vi "TestMain.vi"() -> ()   [LabVIEW 2019]
uses:
  <vilib>/Platform/TimedLoop/XDataNode/timing_clust.ctl
  <vilib>/Platform/TimedLoop/XDataNode/nitl_modes.ctl
  <vilib>/Platform/TimedLoop/XDataNode/wakeup.ctl
  <vilib>/myRIO/Instrument Drivers/Onboard IO/PWM/typedefs/PWM Reference.ctl
  <vilib>/myRIO/Common/Instrument Driver Framework/Utilities/typedefs/myRIO Generic Hardware Reference.ctl
  <vilib>/myRIO/Common/Instrument Driver Framework/Utilities/typedefs/Hardware Version Enum.ctl
  <vilib>/myRIO/Common/Instrument Driver Framework/Utilities/typedefs/myRIO v1.0 Reference.ctl
  <vilib>/myRIO/Common/Instrument Driver Framework/Utilities/typedefs/Generic FPGA Reference.ctl
  <vilib>/myRIO/Common/Instrument Driver Framework/myRIO v1.0/PWM/typedefs/PWM Channels Enum.ctl
  <vilib>/myRIO/Instrument Drivers/Onboard IO/PWM/typedefs/PWM Configuration.ctl
  <vilib>/userDefined/High Color/nirio_resource_hc.ctl
  <vilib>/myRIO/Instrument Drivers/Onboard IO/DIO/typedefs/DIO Reference.ctl
  <vilib>/myRIO/Common/Instrument Driver Framework/myRIO v1.0/DIO/typedefs/DIO Channels List.ctl
  <vilib>/myRIO/Common/Instrument Driver Framework/myRIO v1.0/DIO/typedefs/DIO Channels Enum.ctl
  <vilib>/myRIO/Common/Instrument Driver Framework/Utilities/vis/Is FPGA Ref Available.vi
  <vilib>/myRIO/Common/Instrument Driver Framework/myRIO v1.0/PWM/vis/myRIO v1.1 Open PWM.vi
  <vilib>/myRIO/Instrument Drivers/Onboard IO/PWM/vis/Set Duty Cycle and Frequency.vi
  <vilib>/myRIO/Common/Instrument Driver Framework/myRIO v1.0/DIO/vis/myRIO v1.1 Open DIO.vi
  <extravilib>/ChannelInstances/Tag-bool/Write With Abort.vi
  <extravilib>/ChannelInstances/Tag-bool/Read With Abort.vi
  <vilib>/myRIO/Common/Instrument Driver Framework/Utilities/vis/Validate Channels.vi
  <vilib>/myRIO/Common/Instrument Driver Framework/myRIO v1.0/PWM/vis/myRIO v1.0 Reserve PWM.vi
  <vilib>/myRIO/Common/Instrument Driver Framework/myRIO v1.0/DIO/vis/myRIO v1.0 Reserve DIO.vi
  <vilib>/myRIO/Common/Instrument Driver Framework/myRIO v1.0/I2C/vis/myRIO v1.0 Close I2C.vi
  <vilib>/myRIO/Common/Instrument Driver Framework/myRIO v1.0/UART/vis/myRIO v1.0 Close UART.vi
  <vilib>/myRIO/Common/Instrument Driver Framework/myRIO v1.0/PWM/vis/myRIO v1.0 Build MUX Configuration PWM.vi
  <vilib>/myRIO/Common/Instrument Driver Framework/myRIO v1.0/Resource Manager/vis/myRIO v1.0 Reserve Channel List.vi
  <vilib>/myRIO/Common/Instrument Driver Framework/myRIO v1.0/DIO/vis/myRIO v1.0 Build MUX Configuration DIO.vi
  <vilib>/myRIO/Common/Instrument Driver Framework/myRIO v1.0/I2C/vis/myRIO v1.0 Unreserve I2C.vi
  <vilib>/myRIO/Common/Instrument Driver Framework/myRIO v1.0/Resource Manager/vis/myRIO v1.0 Create Configuration List.vi
  <vilib>/myRIO/Common/Instrument Driver Framework/myRIO v1.0/Resource Manager/vis/myRIO v1.0 Reserve Channel.vi
  <vilib>/myRIO/Common/Instrument Driver Framework/myRIO v1.0/Resource Manager/vis/myRIO v1.0 Unreserve Channel.vi
  <vilib>/myRIO/Common/Instrument Driver Framework/myRIO v1.0/I2C/vis/myRIO v1.0 Build MUX Configuration I2C.vi
  <vilib>/myRIO/Common/Instrument Driver Framework/myRIO v1.0/Resource Manager/vis/myRIO v1.0 Unreserve Channel List.vi
  <vilib>/myRIO/Common/Instrument Driver Framework/myRIO v1.0/Resource Manager/vis/myRIO v1.0 Build Mutex Name.vi
  <extravilib>/ChannelInstances/Tag-bool/Instantiate.vi
  <extravilib>/ChannelInstances/Tag-bool/EndpointRead.vi
  <vilib>/Utility/VariantDataType/GetNumericInfo.vi
  <vilib>/Utility/error.llb/Error Cluster From Error Code.vi
  <vilib>/myRIO/Common/Instrument Driver Framework/myRIO v1.0/myRIO v1.1 Open.vi
  <vilib>/myRIO/Common/Instrument Driver Framework/Utilities/vis/IO Manager.vi
  <vilib>/myRIO/Common/Instrument Driver Framework/Utilities/vis/Configuration Manager.vi
  <vilib>/myRIO/Common/Instrument Driver Framework/myRIO v1.0/Resource Manager/vis/myRIO v1.0 Configure IO.vi
  <vilib>/myRIO/Common/Instrument Driver Framework/myRIO v1.0/myRIO v1.0 Close.vi
  <vilib>/myRIO/Common/Instrument Driver Framework/myRIO v1.0/PWM/vis/myRIO v1.0 Write PWM.vi
  <vilib>/myRIO/Common/Instrument Driver Framework/myRIO v1.0/DIO/vis/myRIO v1.0 Write DIO.vi
  <vilib>/myRIO/Common/Instrument Driver Framework/myRIO v1.0/I2C/vis/myRIO v1.0 Shutdown I2C.vi
  <vilib>/rvi/errors/niLvFpgaAdjustHostInterfaceError.vi
  <vilib>/FPGAPlugInAG/Dynamic/niLvFpga_Abort_Dynamic.vi
  <vilib>/myRIO/Common/Instrument Driver Framework/Utilities/vis/FPGA Ref Manager.vi
  <vilib>/myRIO/Common/Instrument Driver Framework/myRIO v1.0/myRIO v1.0 Reset FPGA.vi
  <vilib>/myRIO/Common/Instrument Driver Framework/myRIO v1.0/IRQ/vis/myRIO v1.0 IRQ Info FGV.vi
  <vilib>/myRIO/Common/Instrument Driver Framework/myRIO v1.0/IRQ/vis/myRIO v1.0 Timer IRQ Info FGV.vi
  <vilib>/myRIO/Common/Instrument Driver Framework/myRIO v1.0/IRQ/vis/myRIO v1.0 ISR Agent.vi
  <vilib>/myRIO/Instrument Drivers/Utilities/vis/Reset Index.vi
  <vilib>/myRIO/Common/Instrument Driver Framework/myRIO v1.0/Resource Manager/vis/myRIO v1.0 Block Write Resource Manager.vi
  <vilib>/FPGAPlugInAG/Dynamic/niLvFpga_Close_Dynamic.vi
  <extravilib>/ChannelInstances/Tag-bool/Endpoint.vi
  <vilib>/platform/TimedLoop/XDataNode/XDataNode.xnode
  <vilib>/myRIO/Express VI/Onboard IO/PWM/PWM Express VI.xnode
  <vilib>/myRIO/Instrument Drivers/Onboard IO/PWM/vis/myRIO PWM Open.xnode
  <vilib>/myRIO/Express VI/Onboard IO/DO/DO Express VI.xnode
  <vilib>/myRIO/Instrument Drivers/Onboard IO/DIO/vis/myRIO DIO Open.xnode
  <vilib>/rvi/interface/nirviReadWriteControl/nirviReadWriteControl.xnode
  <vilib>/rvi/interface/nirviMethod/nirviMethod.xnode
  <vilib>/rvi/interface/nirviCloseFPGA/nirviCloseFPGA.xnode
  <vilib>/rvi/interface/Simulation/niFpgaSimulationCallBeginRW.vi
  <vilib>/Platform/TimedLoop/XDataNode/XDNodeRunTimeDep.lvlib
  <vilib>/myRIO/Instrument Drivers/Utilities/Utilities.lvlib
  NiFpgaLv.dll
  <extravilib>/ChannelInstances/Tag-bool.lvlib
  <vilib>/myRIO/Instrument Drivers/Onboard IO/PWM/PWM.lvlib
  <vilib>/myRIO/Instrument Drivers/Onboard IO/DIO/DIO.lvlib
  <vilib>/myRIO/Instrument Drivers/Onboard IO/I2C/I2C.lvlib
panel:
  in  "Speed (km/h)":dbl
  in  "Test FM only":bool
  in  "Old (F), new (T) PID":bool
  in  "Inner PID T/F":bool
  in  "D_i":dbl
  in  "I_i":dbl
  in  "P_i":dbl
  in  "Log file path":path
  out "Duty Cycle":dbl
  in  "Angle limit":i32
  in  "D_o":dbl
  in  "I_o":dbl
  in  "P_o":dbl
  out "Combined loop duration time (us)":i64
  in  "Loop durations":T1(tab)
  out "IMU Data gathering duration(us)":i64(graph)
  out "Encoder data gathering duration(us)":i64(graph)
  out "Steering Motor duration(us)":i64(graph)
  out "E-Stop loop duration (us)":i64(graph)
  in  "GO":bool
  in  "E-stop":bool
  out "Indicator":bool
  in  "Encoder Position Reset":bool
  out "Encoder Velocity (Counts/Interval)":i32
  out "Encoder Acceleration (Counts/Interval)":i32
  out "Encoder Position (Counts)":i32
  out "IMU Gyro Chart":cluster{dbl, dbl, dbl}(graph)
  out "IMU Acc Chart":cluster{dbl, dbl, dbl}(graph)
  # "Steering Motor"
  # "Forward Motor"
  # "Outer"
  # "Inner"
  # "Start Motors"
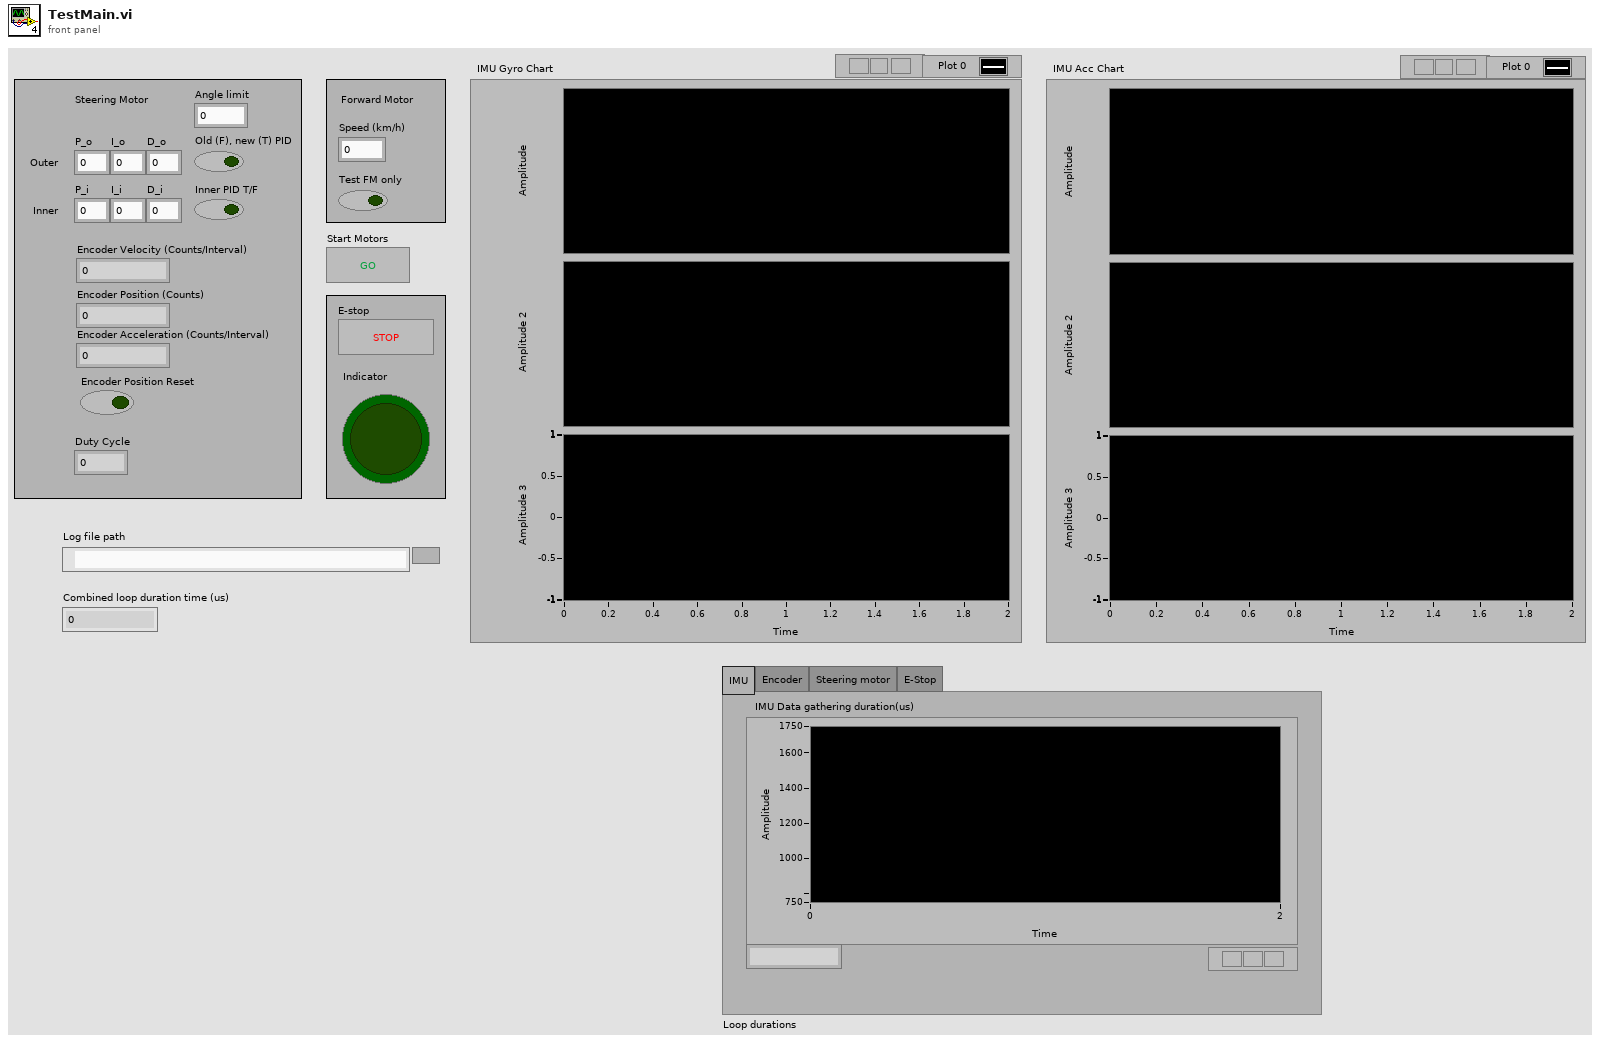
[diagram p1: front panel]
types:
  T1 = enum32{"IMU", "Encoder", "Steering motor", "E-Stop"}
  T2 = enum16{"open", "open or create", "create or replace", "create", "open (read-only)"}
  T3 = typedef "I2C.lvlib/I2C Reference.ctl" = cluster{"myRIO Reference":T4, "I2C Channels Enum":T8, "I2C Configuration":T9}
  T4 = typedef "myRIO Generic Hardware Reference.ctl" = cluster{"myRIO Model":T5, "myRIO Hardware Reference":T6}
  T5 = typedef "Hardware Version Enum.ctl" = enum16{"Unknown", "myRIO-1900", "myRIO-1950", "roboRIO", "NI ELVIS RIO CM", "ELVIS III"}
  T6 = typedef "myRIO v1.0 Reference.ctl" = cluster{"Generic FPGA Reference":T7, "Allow multiple opens":bool}
  T7 = typedef "Generic FPGA Reference.ctl" = refnum<k20>
  T8 = typedef "I2C Channels Enum.ctl" = enum16{"Not Connected", "A/I2C", "B/I2C", "I2C/I2C"}
  T9 = typedef "I2C.lvlib/I2C Configuration.ctl" = cluster{"I2C Transfer Rate":T10}
  T10 = typedef "I2C.lvlib/I2C Transfer Rate.ctl" = enum16{"Standard mode (100 kbps)", "Fast mode (400 kbps)"}
  T11 = typedef "XDNodeRunTimeDep.lvlib/timing_clust.ctl" = cluster{"Expected End [f-1]":u64, "Actual End [f-1]":u64, "Finished Late? [f-1]":bool, "Expected End [i-1]":u64, "Actual End [i-1]":u64, "Finished Late? [i-1]":bool, "Expected Start [i]":u64, "Actual Start [i]":u64, "Expected Start [f]":u64, "Actual Start [f]":u64, "Source Name":string, "Structure Name":string, "Period":i64, "Deadline":i64, "Offset":i64, "Start":i64, "Priority":i32, "Timeout":i32, "Mode":T12, "Wakeup Reason":T13, "Error":errorcluster, "Source Type":string, "Secondary Source Type":string, "Global End Time":u64, "Global Start Time":u64, "Frame Duration":u64, "Iteration Duration":u64, "Assigned CPU":i32, "I/O Scan Engine Mode":u32}
  T12 = typedef "XDNodeRunTimeDep.lvlib/nitl_modes.ctl" = enum32{"No Change", "Process missed periods, maintain original phase", "Discard missed periods, maintain original phase", "Process missed periods, ignore original phase", "Discard missed periods, ignore original phase"}
  T13 = typedef "XDNodeRunTimeDep.lvlib/wakeup.ctl" = enum32{"Normal", "Aborted", "Asynchronous wakeup", "Timing source error", "Timed loop error", "Timeout"}
  T14 = typedef "Tag-bool.lvlib/))Channel.ctl" = refnum<queue>
  T15 = typedef "PWM.lvlib/PWM Reference.ctl" = cluster{"myRIO Reference":T4, "PWM Channels Enum":T16, "PWM Configuration":T17}
  T16 = typedef "PWM Channels Enum.ctl" = enum16{"Not Connected", "C/PWM0", "C/PWM1", "A/PWM0", "A/PWM1", "A/PWM2", "A/PWM3", "A/PWM4", "A/PWM5", "A/PWM6", "A/PWM7", "A/PWM8", "A/PWM9", "A/PWM10", "A/PWM11", "A/PWM12", "A/PWM13", "A/PWM14", "A/PWM15", "A/PWM16", "A/PWM17", "A/PWM18", "A/PWM19", "B/PWM0", "B/PWM1", "B/PWM2", "B/PWM3", "B/PWM4", "B/PWM5", "B/PWM6", "B/PWM7", "B/PWM8", "B/PWM9", "B/PWM10", "B/PWM11", "B/PWM12", "B/PWM13", "B/PWM14", "B/PWM15", "B/PWM16", "B/PWM17", "B/PWM18", "B/PWM19", "PWM/PWM0", "PWM/PWM1", "PWM/PWM2", "PWM/PWM3", "PWM/PWM4", "PWM/PWM5", "PWM/PWM6", "PWM/PWM7", "PWM/PWM8", "PWM/PWM9"}
  T17 = typedef "PWM.lvlib/PWM Configuration.ctl" = cluster{"Frequency":dbl, "Duty Cycle":dbl}
  T18 = typedef "nirio_resource_hc.ctl" = tag
  T19 = typedef "DIO.lvlib/DIO Reference.ctl" = cluster{"myRIO Reference":T4, "DIO Channels List":T20}
  T20 = typedef "DIO Channels List.ctl" = T21[]
  T21 = typedef "DIO Channels Enum.ctl" = enum16{"Not Connected", "C/DIO0", "C/DIO1", "C/DIO2", "C/DIO3", "C/DIO4", "C/DIO5", "C/DIO6", "C/DIO7", "A/DIO0", "A/DIO1", "A/DIO2", "A/DIO3", "A/DIO4", "A/DIO5", "A/DIO6", "A/DIO7", "A/DIO8", "A/DIO9", "A/DIO10", "A/DIO11", "A/DIO12", "A/DIO13", "A/DIO14", "A/DIO15", "A/DIO16", "A/DIO17", "A/DIO18", "A/DIO19", "B/DIO0", "B/DIO1", "B/DIO2", "B/DIO3", "B/DIO4", "B/DIO5", "B/DIO6", "B/DIO7", "B/DIO8", "B/DIO9", "B/DIO10", "B/DIO11", "B/DIO12", "B/DIO13", "B/DIO14", "B/DIO15", "B/DIO16", "B/DIO17", "B/DIO18", "B/DIO19", "LED0", "LED1", "LED2", "LED3", "Button0", "DIO/DIO0", "DIO/DIO1", "DIO/DIO2", "DIO/DIO3", "DIO/DIO4", "DIO/DIO5", "DIO/DIO6", "DIO/DIO7", "DIO/DIO8", "DIO/DIO9", "SPI/CS0", "SPI/CS1", "SPI/CS2", "SPI/CS3", "LED RADIO (Green)", "LED RADIO (Red)", "LED COMM (Green)", "LED COMM (Red)", "LED MODE (Green)", "LED MODE (Red)"}
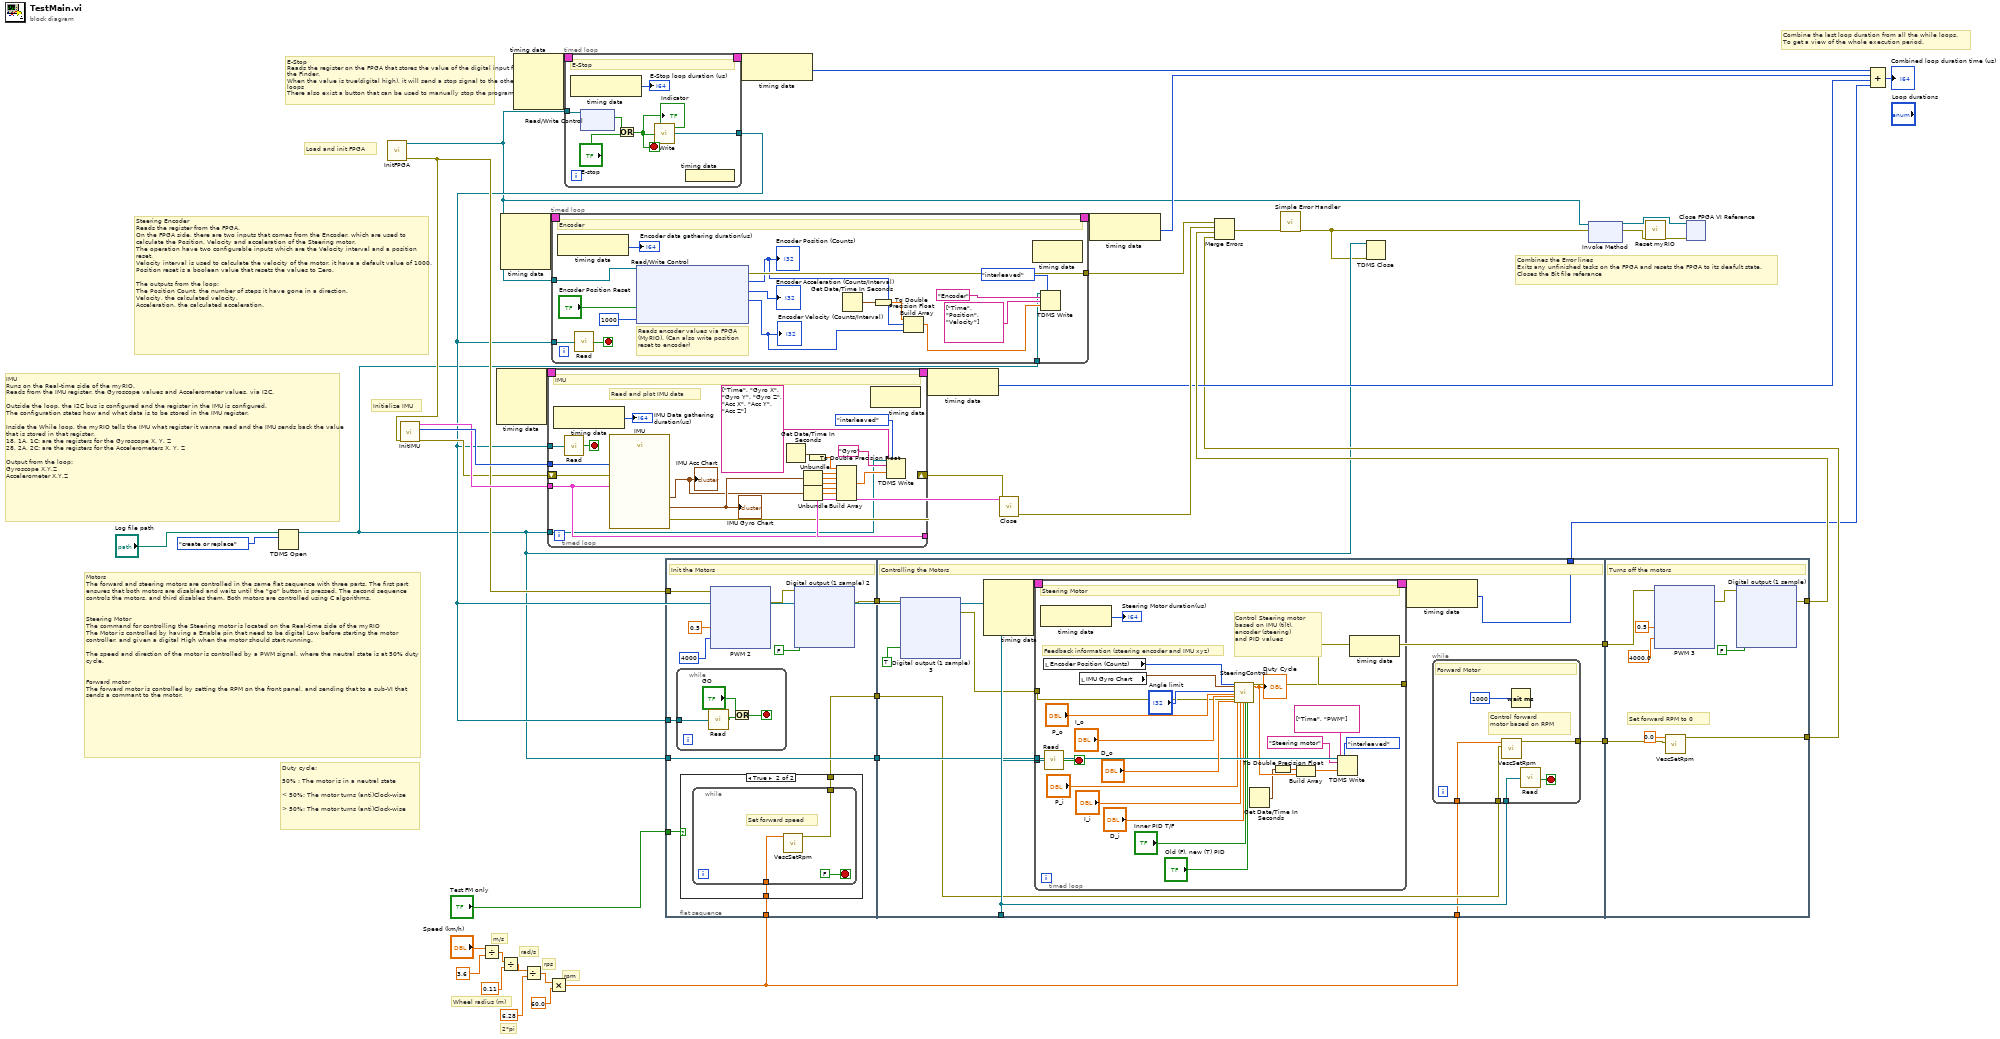
[diagram p0: block diagram]
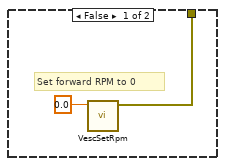
[diagram p2: hidden frame]
diagram:
  # "2*pi"
  # "rpm"
  # "rps"
  # "rad/s"
  # "Wheel radius (m)"
  # "m/s"
  # "Duty cycle:\n\n50% : The motor is in a neutral state\n\n< 50%: The motor turns (anti)Clock-wise\n\n> 50%: The motor turns (anti)Clock-wise"
  # "Initialize IMU"
  # "Load and init FPGA"
  # "Combines the Error lines\nExits any unfinished tasks on the FPGA and resets the FPGA to its deafult state.\nCloses the Bit file referance"
  # "Combine the last loop duration from all the while loops.\nTo get a view of the whole execution period."
  # "Motors\nThe forward and steering motors are controlled in the same flat sequence with three parts. The first part ensures that both motors are disabled and waits until the \"go\" button is pressed. The second sequence controls the motors, and third disables them. Both motors are controlled using C algorithms.\n\n\nSteering Motor\nThe command for controlling the Steering motor is located on the Real-time side of the myRIO\nThe Motor is controlled by having a Enable pin that need to be digital Low before starting the motor controller, and given a digital High when the motor should start running.\n\nThe speed and direction of the motor is controlled by a PWM signal, where the neutral state is at 50% duty cycle.\n\n\nForward motor\nThe forward motor is controlled by setting the RPM on the front panel, and sending that to a sub-VI that sends a commant to the motor."
  # "IMU\nRuns on the Real-time side of the myRIO.\nReads from the IMU register, the Gyroscope values and Accelerometer values, via I2C.\n\nOutside the loop, the I2C bus is configured and the register in the IMU is configured.\nThe configuration states how and what data is to be stored in the IMU register.\n\nInside the While loop, the myRIO tells the IMU what register it wanna read and the IMU sends back the value that is stored in that register.\n18, 1A, 1C: are the registers for the Gyroscope X, Y, Z\n28, 2A, 2C: are the registers for the Accelerometers X, Y, Z\n\nOutput from the loop:\nGyroscope X,Y,Z\nAccelerometer X,Y,Z"
  # "Steering Encoder\nReads the register from the FPGA. \nOn the FPGA side, there are two inputs that comes from the Encoder, which are used to calculate the Position, Velocity and acceleration of the Steering motor.\nThe operation have two configurable inputs which are the Velocity interval and a position reset.\nVelocity interval is used to calculate the velocity of the motor, it have a default value of 1000.\nPosition reset is a boolean value that resets the values to Zero.\n\nThe outputs from the loop:\nThe Position Count, the number of steps it have gone in a direction. \nVelocity, the calculated velocity.\nAcceleration, the calculated acceleration."
  # "E-Stop\nReads the register on the FPGA that stores the value of the digital input from the Finder.\nWhen the value is true(digital high), it will send a stop signal to the other while loops\nThere also exist a button that can be used to manually stop the program."
  n1 = TDMS Open(10:T2."create or replace" ("operation (0:open)"), 11:"Log file path") -> (3:w15:refnum<k34>)  [unwired: 5 in, 1 out]
  n2 = call "InitFPGA.vi"() -> ("error out"=w30:errorcluster, "Refnum out"=w11:refnum<k20>)  [unwired: 10 in]
  n3 = call "InitIMU.vi"("error in (no error)"=w30) -> ("error out"=w25:errorcluster, "Acc/Gyro  address"=w32:u8, "I2C Ref Out"=w31:T3)  [unwired: 8 in]
  n4 = Divide(x="Speed (km/h)", y=3.6) -> (x/y=w7:dbl)
  n5 = node-c288() -> (w39:T11)  [unwired: 4 in]
  n6 = node-c288() -> (w43:T11)  [unwired: 4 in]
  n7 = Divide(x=w7, y=0.11) -> (x/y=w5:dbl)
  n8 = node-c288() -> (w37:T11)  [unwired: 4 in]
  n9 = Divide(x=w5, y=6.28) -> (x/y=w4:dbl)
  n10 = Multiply(x=w4, y=60.0) -> (x*y=w1:dbl)
  n11 = timed-loop {
    timing: w37 -> [_]
    timing-out: [_] -> w36
    tunnel: w11 -> [w52]
    tunnel: [w51] -> w23
    stop <- w47 stop-if-true
    # "E-Stop"
    n12 = node-c288() -> (→"E-Stop loop duration (us)":i64)  [unwired: 1 in]
    n13 = xnode "Read/Write Control"("FPGA VI Reference In"=w52) -> ("E-Stop"=w50:bool)  [unwired: 1 in, 2 out]
    n14 = Or(x=w50, y="E-stop") -> (x .or. y?=w47:bool)
    "Indicator" <- w47
    n15 = call <vilib>:"Write.vi"("element"=w47) -> ("channel"=w51:T14)  [unwired: 1 out]
    n16 = node-c288() -> ()  [unwired: 1 out]
  }
  n17 = timed-loop {
    timing: w39 -> [_]
    timing-out: [_] -> w38
    tunnel: w32 -> [w77]
    tunnel: w31 -> [w74]
    shift-right: [w71] -> w26
    shift-left: w25 -> [w76]
    tunnel: [w74] -> w29
    tunnel: w23 -> [w73]
    tunnel: w15 -> [w66]
    stop <- w72 stop-if-true
    # "Read and plot IMU data"
    # "IMU"
    n18 = node-c288() -> (→"IMU Data gathering duration(us)":i64)  [unwired: 1 in]
    n19 = call <extravilib>:"Read.vi"("channel"=w73) -> ("element"=w72:bool)  [unwired: 1 in, 1 out]
    n20 = call "IMU.vi"("error in (no error)"=w76, "Acc/Gyro  address"=w77, "I2C Ref"=w74) -> ("error out"=w71:errorcluster, "IMU Acc"=w59:cluster{dbl, dbl, dbl}, "IMU Gyro"=w70:cluster{dbl, dbl, dbl})  [unwired: 6 in]
    "IMU Acc Chart" <- w59
    "IMU Gyro Chart" <- w70
    n21 = Get Date/Time In Seconds() -> (seconds since 1Jan1904=w64:timestamp)
    n22 = Unbundle(w70) -> (w69:dbl, w61:dbl, w60:dbl)
    n23 = Unbundle(w59) -> (w58:dbl, w57:dbl, w56:dbl)
    n24 = To Double Precision Float(number=w64) -> (double precision float=w65:dbl)
    n25 = Build Array(w65, w69, w61, w60, w58, w57, w56) -> (w67:dbl[])
    n26 = node-c288() -> ()  [unwired: 1 in, 1 out]
    n27 = TDMS Write(0:w66, 1:enum16{"decimated", "interleaved"}."interleaved" ("data layout (0:decimated)"), 5:"Gyro" ("group name in (Untitled)"), 7:string[] ["Time", "Gyro X", "Gyro Y", "Gyro Z", "Acc X", "Acc Y", "Acc Z"] ("channel name(s) in (Untitled)"), 9:w67) -> ()  [unwired: 1 in, 4 out]
  }
  n28 = timed-loop {
    timing: w43 -> [_]
    timing-out: [_] -> w42
    tunnel: w11 -> [w97]
    tunnel: [w96] -> w41
    tunnel: w23 -> [w91]
    tunnel: w15 -> [w84]
    stop <- w90 stop-if-true
    # "Reads encoder values via FPGA\n(MyRIO). (Can also write position\nreset to encoder)"
    # "Encoder"
    n29 = node-c288() -> (→"Encoder data gathering duration(us)":i64)  [unwired: 1 in]
    n30 = call <extravilib>:"Read.vi"("channel"=w91) -> ("element"=w90:bool)  [unwired: 1 in, 1 out]
    n31 = xnode "Read/Write Control"("FPGA VI Reference In"=w97, "Position Reset"="Encoder Position Reset", "Velocity Interval (uSec)"=u32 1000) -> ("error out"=w96:errorcluster, "Position (Counts)"=w87:i32, "Acceleration (Counts/Interval)"=→"Encoder Acceleration (Counts/Interval)":i32, "Velocity (Counts/Interval)"=w86:i32)  [unwired: 1 in, 1 out]
    "Encoder Position (Counts)" <- w87
    "Encoder Velocity (Counts/Interval)" <- w86
    n32 = Get Date/Time In Seconds() -> (seconds since 1Jan1904=w82:timestamp)
    n33 = To Double Precision Float(number=w82) -> (double precision float=w83:dbl)
    n34 = Build Array(w83, w87, w86) -> (w85:dbl[])
    n35 = node-c288() -> ()  [unwired: 1 in, 1 out]
    n36 = TDMS Write(0:w84, 1:enum16{"decimated", "interleaved"}."interleaved" ("data layout (0:decimated)"), 5:"Encoder" ("group name in (Untitled)"), 7:string[] ["Time", "Position", "Velocity"] ("channel name(s) in (Untitled)"), 9:w85) -> ()  [unwired: 1 in, 4 out]
  }
  n37 = flat-sequence {
    tunnel: [w110] -> w35
    tunnel: w30 -> [w108]
    tunnel: w23 -> [w105]
    tunnel: [w101] -> w22
    tunnel: w15 -> [w104]
    tunnel: [w104] -> w16
    tunnel: "Test FM only" -> [w103]
    tunnel: w1 -> [w102]
    tunnel: w35 -> [w204]
    tunnel: [w201] -> w13
    tunnel: w23 -> [w198]
    tunnel: w22 -> [w194]
    tunnel: [w197] -> w21
    tunnel: [w196] -> w19
    tunnel: w16 -> [w195]
    tunnel: w1 -> [w193]
    tunnel: [w283] -> w27
    tunnel: w21 -> [w278]
    tunnel: [w277] -> w20
    tunnel: w19 -> [w276]
    frame #0 {
      # "Init the Motors"
      n38 = while {
        tunnel: w105 -> [w119]
        stop <- w122 stop-if-true
        n39 = call <extravilib>:"Read.vi"("channel"=w119) -> ("element"=w120:bool)  [unwired: 1 in, 1 out]
        n40 = Or(x="GO", y=w120) -> (x .or. y?=w122:bool)
      }
      n41 = case shown="True" w103 {
        tunnel: w102 -> [_ w115]
        tunnel: [w112 w114] -> w101
        frame False {
          # "Set forward RPM to 0"
          n42 = call "VescSetRpm.vi"("Speed (rpm)"=0.0) -> ("error out"=w112:errorcluster)  [unwired: 10 in]
        }
        frame True {
          n43 = while {
            tunnel: w115 -> [w118]
            tunnel: [w116] -> w114
            stop <- FALSE stop-if-true
            # "Set forward speed"
            n44 = call "VescSetRpm.vi"("Speed (rpm)"=w118) -> ("error out"=w116:errorcluster)  [unwired: 10 in]
          }
        }
      }
      n45 = xnode "PWM 2"("Duty Cycle"=0.5, "Frequency [Hz]"=4000, "error in (no error)"=w108) -> ("error out"=w111:errorcluster)
      n46 = xnode "Digital output (1 sample) 2"("B/DIO4 (Pin 19)"=FALSE ("B/DIO1 (Pin 13)"), "error in (no error)"=w111) -> ("error out"=w110:errorcluster)
    }
    frame #1 {
      # "Controlling the Motors"
      n47 = xnode "Digital output (1 sample) 3"("B/DIO4 (Pin 19)"=TRUE ("B/DIO1 (Pin 13)"), "error in (no error)"=w204) -> ("error out"=w200:errorcluster)
      n48 = node-c288() -> (w203:T11)  [unwired: 4 in]
      n49 = timed-loop {
        tunnel: w200 -> [w225]
        timing: w203 -> [_]
        timing-out: [_] -> w202
        tunnel: w198 -> [w227]
        tunnel: [w224] -> w196
        tunnel: w195 -> [w223]
        stop <- w234 stop-if-true
        # "Feedback information (steering encoder and IMU xyz)"
        # "Control Steering motor\nbased on IMU (tilt), \nencoder (steering)\nand PID values"
        # "Steering Motor"
        n50 = node-c288() -> (→"Steering Motor duration(us)":i64)  [unwired: 1 in]
        n51 = local read "Encoder Position (Counts)"() -> (w231:i32)
        n52 = call <extravilib>:"Read.vi"("channel"=w227) -> ("element"=w234:bool)  [unwired: 1 in, 1 out]
        n53 = local read "IMU Gyro Chart"() -> (w232:cluster{dbl, dbl, dbl})
        n54 = call "SteeringControl.vi"("Position (Counts)"=w231, "Cluster"=w232, "Limit"="Angle limit", "P_o gain"="P_o", "I_o gain"="I_o", "error in (no error)"=w225, "D_o gain"="D_o", "P_i gain"="P_i", "I_i gain"="I_i", "D_i gain"="D_i", "Inner PID T/F"="Inner PID T/F", "Old (F), new (T) PID"="Old (F), new (T) PID") -> ("error out"=w224:errorcluster, "PWM Out"=w220:dbl)  [unwired: 14 in]
        "Duty Cycle" <- w220
        n55 = Get Date/Time In Seconds() -> (seconds since 1Jan1904=w218:timestamp)
        n56 = To Double Precision Float(number=w218) -> (double precision float=w219:dbl)
        n57 = Build Array(w219, w220) -> (w221:dbl[])
        n58 = TDMS Write(0:w223, 1:enum16{"decimated", "interleaved"}."interleaved" ("data layout (0:decimated)"), 5:"Steering motor" ("group name in (Untitled)"), 7:string[] ["Time", "PWM"] ("channel name(s) in (Untitled)"), 9:w221) -> ()  [unwired: 1 in, 4 out]
        n59 = node-c288() -> ()  [unwired: 1 in, 1 out]
      }
      n60 = node-c288(w202) -> (w201:i64)
      n61 = while "Timed Loop" {
        tunnel: w198 -> [w209]
        tunnel: w194 -> [w207]
        tunnel: [w206] -> w197
        tunnel: w193 -> [w205]
        stop <- w210 stop-if-true
        # "Control forward\nmotor based on RPM"
        # "Forward Motor"
        n62 = call "VescSetRpm.vi"("error in (no error)"=w207, "Speed (rpm)"=w205) -> ("error out"=w206:errorcluster)  [unwired: 9 in]
        n63 = Wait (ms)(milliseconds to wait=1000) -> ()  [unwired: 1 out]
        n64 = call <extravilib>:"Read.vi"("channel"=w209) -> ("element"=w210:bool)  [unwired: 1 in, 1 out]
      }
    }
    frame #2 {
      # "Set forward RPM to 0"
      # "Turns off the motors"
      n65 = xnode "PWM 3"("Duty Cycle"=0.5, "Frequency [Hz]"=4000.0, "error in (no error)"=w276) -> ("error out"=w280:errorcluster)
      n66 = call "VescSetRpm.vi"("error in (no error)"=w278, "Speed (rpm)"=0.0) -> ("error out"=w277:errorcluster)  [unwired: 9 in]
      n67 = xnode "Digital output (1 sample)"("B/DIO4 (Pin 19)"=FALSE ("B/DIO1 (Pin 13)"), "error in (no error)"=w280) -> ("error out"=w283:errorcluster)
    }
  }
  n68 = node-c288(w36) -> (w12:i64)
  n69 = node-c288(w38) -> (w24:i64)
  n70 = call <vilib>:"Close.vi"("error in (no error)"=w26, "I2C Ref In"=w29) -> ("error out"=w28:errorcluster)  [unwired: 9 in]
  n71 = node-c288(w42) -> (w34:i64)
  n72 = Merge Errors(w41, w28, w27, w20) -> (w40:errorcluster)
  n73 = call <vilib>:"Simple Error Handler.vi"("error in (no error)"=w40) -> ("error out"=w14:errorcluster)  [unwired: 4 in, 4 out]
  n74 = TDMS Close(8:w14, 11:w15) -> ()  [unwired: 2 out]
  n75 = xnode "Invoke Method"("FPGA VI Reference In"=w11, "error in"=w14) -> ("FPGA VI Reference Out"=w46:refnum<k20>, "error out"=w44:errorcluster)
  n76 = call <vilib>:"Reset myRIO.vi"("error in (no error)"=w44) -> ("error out"=w45:errorcluster)  [unwired: 10 in]
  n77 = xnode "Close FPGA VI Reference"("FPGA VI Reference In"=w46, "error in"=w45) -> ()  [unwired: 1 out]
  n78 = Compound Arithmetic op=ADD(w12, w34, w24, w13) -> (→"Combined loop duration time (us)":i64)
